vi "TSM Get Speaker AO Settings.vi"(0 "TSM context":T1, 11 "error in (no error)":errorcluster) -> (4 "TSM context Out":T1, 6 "Sampling Rate (Hz)":dbl format="%#_13g", 8 "Samples per channel":i32=1000, 10 "Range (V)":dbl format="%#_13g", 15 "error out":errorcluster)   [LabVIEW 2020]
doc: "Get the DAQmx Analog Output settings of the Speaker from the spec sheet using TSM context"
uses:
  <vilib>/NI_TestStand_SemiconductorModule/NI_TestStand_Semiconductor_Module.lvlibp/PinMap/General/SemiconductorModuleContext.ctl
  <vilib>/NI_TestStand_SemiconductorModule/NI_TestStand_Semiconductor_Module.lvlibp/PinMap/Specs/NamespacedSymbolsToValues.vi
  <vilib>/NI_TestStand_SemiconductorModule/NI_TestStand_Semiconductor_Module.lvlibp
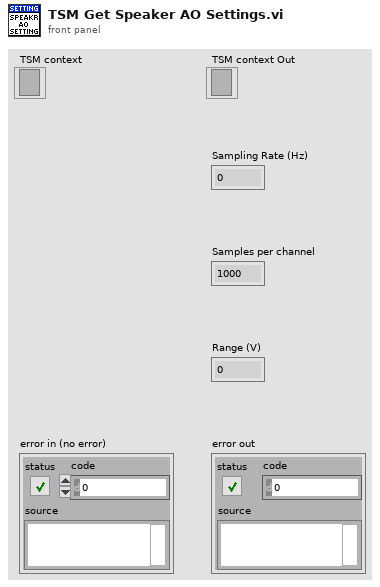
[diagram p1: front panel]
types:
  T1 = typedef "NI_TestStand_Semiconductor_Module.lvlibp/SemiconductorModuleContext.ctl" = refnum<k7>
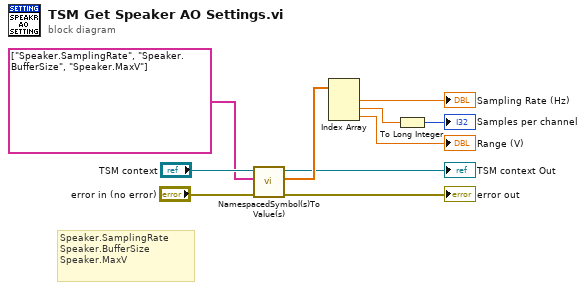
[diagram p0: block diagram]
diagram:
  # "Speaker.SamplingRate\nSpeaker.BufferSize\nSpeaker.MaxV"
  n1 = call-poly <vilib>:"NamespacedSymbol(s)ToValue(s).vi"("error in (no error)"="error in (no error)", "Symbols"=tag[] ["Speaker.SamplingRate", "Speaker.BufferSize", "Speaker.MaxV"], "Semiconductor Module Context"="TSM context") -> ("error out"=→"error out":errorcluster, "Values"=w7:dbl[], "Semiconductor Module Context Out"=→"TSM context Out":T1)  [unwired: 6 in]
  n2 = Index Array(array=w7) -> (element #1=→"Sampling Rate (Hz)":dbl, element #2=w1:dbl, element #3=→"Range (V)":dbl)  [unwired: 3 in]
  n3 = To Long Integer(number=w1) -> (32bit integer=→"Samples per channel":i32)
